vi "sub parse frame title.vi"(8 "error in (no error)":errorcluster, 11 "String":string="<f 20 normal_weapon_atck") -> (0 "error out":errorcluster, 3 "frame title":T1)   [LabVIEW 2018, in "Frame Analizer.lvclass"]
uses:
  Frame Analizer.lvclass
  frame title.ctl
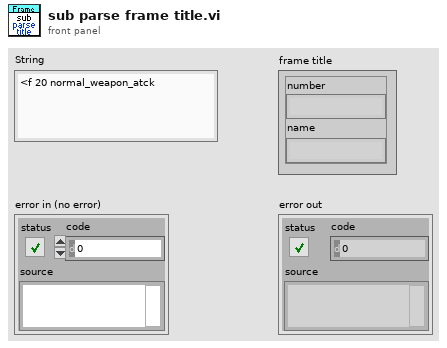
[diagram p1: front panel]
types:
  T1 = typedef "Frame Analizer.lvclass/frame title.ctl" = cluster{"number":string, "name":string}
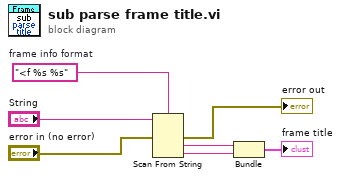
[diagram p0: block diagram]
diagram:
  w7 = "<f %s %s"  # frame info format
  n1 = Scan From String(format string=w7, input string="String", error in="error in (no error)") -> (error out=→"error out":errorcluster, output 1=w5:string, output 2=w4:string)  [unwired: 3 in, 2 out]
  n2 = Bundle(w5, w4) -> (→"frame title":cluster{string, string})  [unwired: 1 in]
